vi "GetSettingsRef.vi"(8 "error in (no error)":errorcluster, 11 "FpgaRefBase in":refnum<class "FpgaRefBase.lvclass">) -> (0 "error out":errorcluster, 2 "Settings FPGA ref":T1, 3 "FpgaRefBase out":refnum<class "FpgaRefBase.lvclass">)   [LabVIEW 2018, in "FpgaRefBase.lvclass"]
uses:
  FpgaRefBase.lvclass
  Scope/controls/settingsFPGAref.ctl
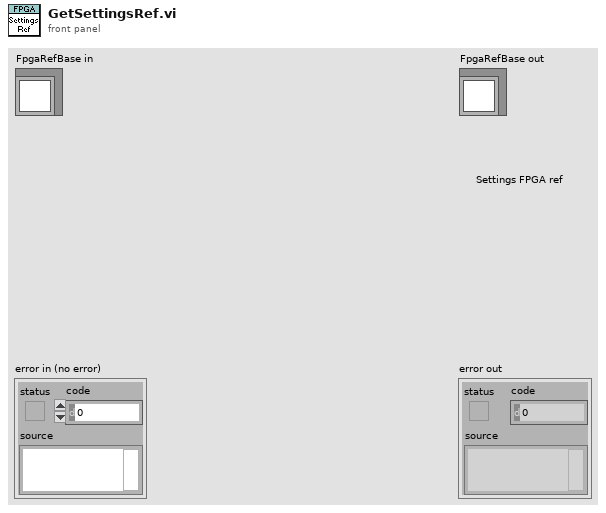
[diagram p1: front panel]
types:
  T1 = typedef "settingsFPGAref.ctl" = refnum<k20>
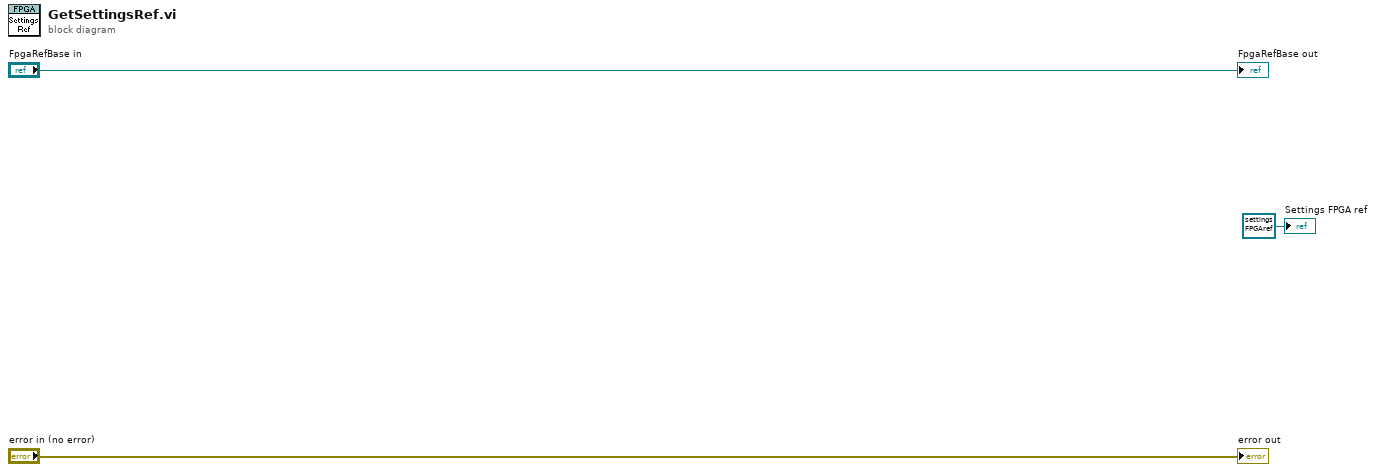
[diagram p0: block diagram]
diagram:
  "error out" <- "error in (no error)"
  "FpgaRefBase out" <- "FpgaRefBase in"
  "Settings FPGA ref" <- T1 refnum ("Settings FPGA ref")
